vi "Retrieve trace.vi"(5 "max points":i32, 7 "Data.PG in":refnum<class "Data.PG.lvclass">, 8 "error in (no error)":errorcluster, 9 "path table:column":string, 10 "End":timestamp, 11 "Start":timestamp) -> (0 "error out":errorcluster, 1 "Column (units)":string, 2 "Trace":cluster{timestamp[], dbl[]}, 3 "Data.PG out":refnum<class "Data.PG.lvclass">)   [LabVIEW 2020, in "Data.PG.lvclass"]
uses:
  Data.PG.lvclass
  <vilib>/Utility/error.llb/Error Cluster From Error Code.vi
  <vilib>/ErrorRing/Error Ring.xnode
panel:
  out "resulting string":string
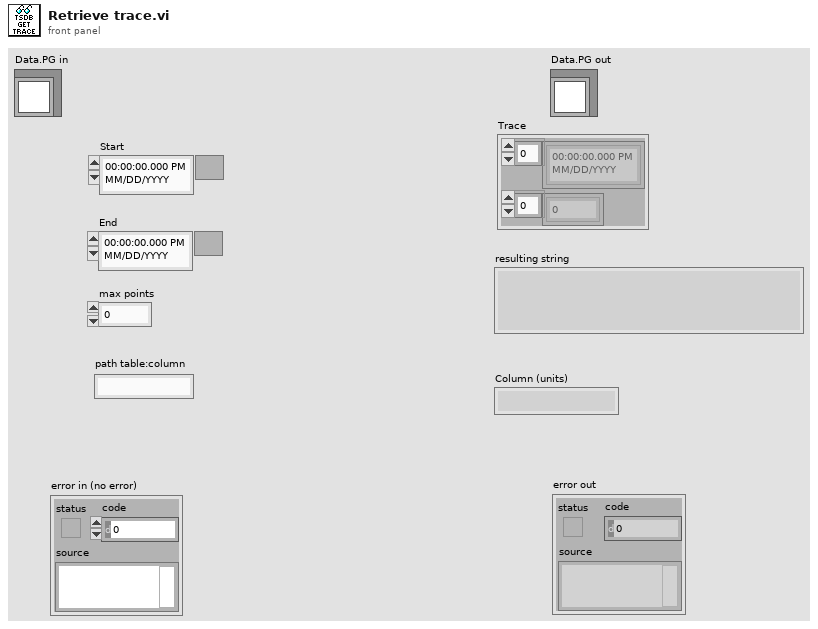
[diagram p1: front panel]
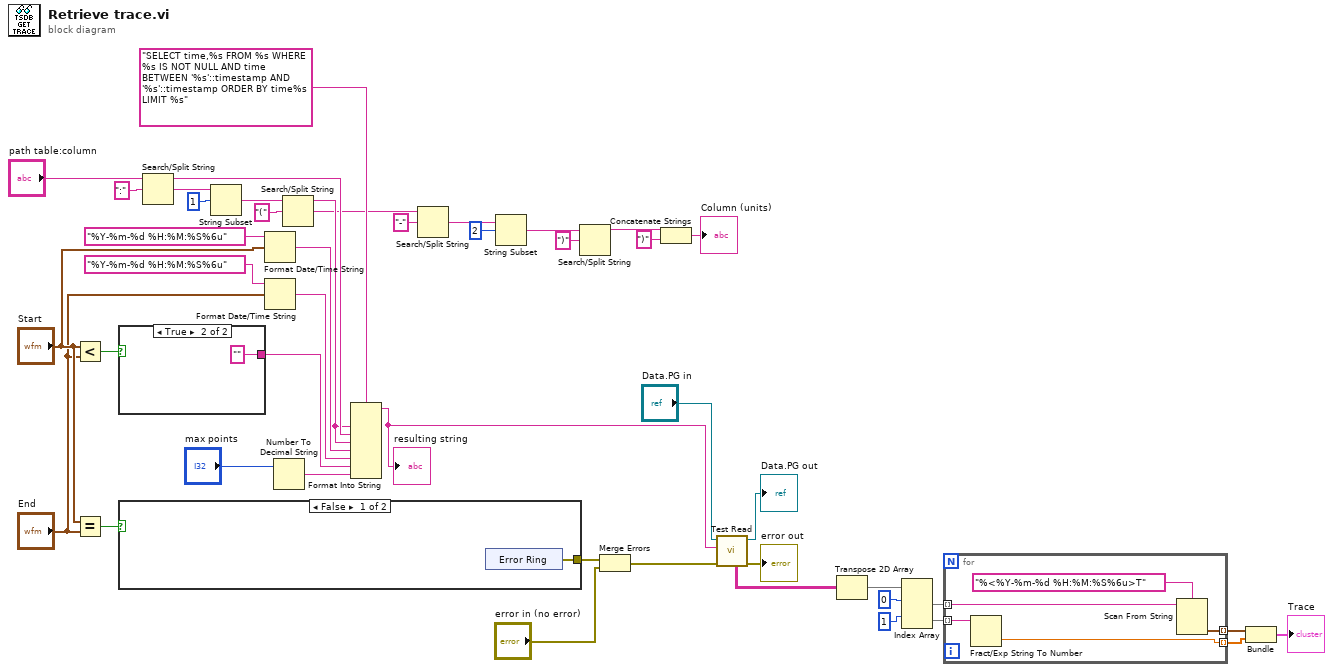
[diagram p0: block diagram]
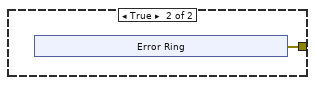
[diagram p2: hidden frame]
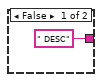
[diagram p3: hidden frame]
diagram:
  n1 = Less?(x="Start", y="End") -> (x < y?=w42:bool)
  n2 = Equal?(x="Start", y="End") -> (x = y?=w41:bool)
  n3 = case shown="True" w42 {
    tunnel: [" DESC" ""] -> w20
    frame False {
    }
    frame True {
    }
  }
  n4 = case shown="False" w41 {
    tunnel: [w48 w50] -> w40
    frame False {
      n5 = xnode "Error Ring"() -> ("error out"=w48:errorcluster)
    }
    frame True {
      n6 = xnode "Error Ring"() -> ("error out"=w50:errorcluster)
    }
  }
  n7 = Search/Split String(string="path table:column", search string/char (-)=":") -> (substring before match=w11:string, match + rest of string=w15:string)  [unwired: 1 in, 1 out]
  n8 = String Subset(string=w15, offset (0)=1) -> (substring=w13:string)  [unwired: 1 in]
  n9 = Format Date/Time String(time format string (%c)="%Y-%m-%d %H:%M:%S%6u", seconds (now)="Start") -> (date/time string=w18:string)  [unwired: 1 in]
  n10 = Format Date/Time String(time format string (%c)="%Y-%m-%d %H:%M:%S%6u", seconds (now)="End") -> (date/time string=w19:string)  [unwired: 1 in]
  n11 = Number To Decimal String(number="max points") -> (decimal integer string=w21:string)  [unwired: 1 in]
  n12 = Search/Split String(string=w13, search string/char (-)="(") -> (substring before match=w10:string, match + rest of string=w9:string)  [unwired: 1 in, 1 out]
  n13 = Format Into String(format string="SELECT time,%s FROM %s WHERE %s IS NOT NULL AND time BETWEEN '%s'::timestamp AND '%s'::timestamp ORDER BY time%s LIMIT %s", w10, w11, w10, w18, w19, w20, w21) -> (resulting string=w22:string)  [unwired: 2 in, 1 out]
  "resulting string" <- w22
  n14 = Search/Split String(string=w9, search string/char (-)="-") -> (match + rest of string=w7:string)  [unwired: 1 in, 2 out]
  n15 = String Subset(string=w7, offset (0)=2) -> (substring=w5:string)  [unwired: 1 in]
  n16 = Search/Split String(string=w5, search string/char (-)=")") -> (substring before match=w3:string)  [unwired: 1 in, 2 out]
  n17 = Merge Errors(w40, "error in (no error)") -> (w38:errorcluster)
  n18 = Concatenate Strings(w3, ")" ("string")) -> (→"Column (units)":string)
  n19 = call-dynamic "Test Read.vi"("error in (no error)"=w38, "command"=w22, "Data.PG in"="Data.PG in") -> ("error out"=→"error out":errorcluster, "Data.PG out"=→"Data.PG out":refnum<class "Data.PG.lvclass">, "Result"=w37:string[][])  [unwired: 3 in, 3 out]
  n20 = Transpose 2D Array(2D array=w37) -> (transposed array=w36:string[][])
  n21 = Index Array(array=w36, index (row) #1=0 ("index (row)"), index (row) #2=1 ("index (row)")) -> (element #1=w33:string[], element #2=w32:string[])  [unwired: 2 in]
  n22 = for {
    tunnel: w33 -> [w59] mode=indexing
    tunnel: w32 -> [w58] mode=indexing
    tunnel: [w57] -> w30 mode=indexing
    tunnel: [w56] -> w31 mode=indexing
    n23 = Fract/Exp String To Number(string=w58) -> (number=w57:dbl)  [unwired: 3 in, 1 out]
    n24 = Scan From String(format string="%<%Y-%m-%d %H:%M:%S%6u>T", input string=w59) -> (output 1=w56:timestamp)  [unwired: 3 in, 3 out]
  }
  n25 = Bundle(w31, w30) -> (→"Trace":cluster{timestamp[], dbl[]})  [unwired: 1 in]
